vi "Send Initialize DLS Laser.vi"(4 "Fault?":bool, 5 "DLS Status LEDs Refnum":refnum<vi>, 6 "DLS Laser ID (A,B,C or D)":enum16{"A", "B", "C", "D"}(ring), 7 "Priority":T1=enum."Normal" caption="Message Priority (Normal)", 8 "error in (no error)":errorcluster, 9 "DLS Range Refnum":refnum<vi>, 10 "DLS COM Port":refnum<visa-resource-name>, 11 "Message Enqueuer in":refnum<class "Message Enqueuer.lvclass">) -> (0 "error out":errorcluster, 3 "Message Enqueuer out":refnum<class "Message Enqueuer.lvclass">)   [LabVIEW 2018, in "FLS Laser Actor.lvlib" / "Initialize FLS Laser Msg.lvclass"]
doc: "Sends the <b>DLS Laser Actor.lvlib:Initialize DLS Laser Msg.lvclass</b> message.\n\nThis message will call <b>Initialize DLS Laser.vi</b> on the <b>DLS Laser Actor.lvlib:DLS Laser Actor.lvclass</b> actor.\n\n<b>Initialize DLS Laser.vi Description</b>"
uses:
  Initialize FLS Laser Msg.lvclass
  <vilib>/ActorFramework/Message Enqueuer/Message Enqueuer.lvclass
  <vilib>/ActorFramework/Message Enqueuer/Message Priority.ctl
  C:/Program Files (x86)/National Instruments/LabVIEW 2018/vi.lib/ActorFramework/Message/Message.lvclass
  Initialize FLS Laser Msg.lvclass/Initialize FLS Laser Msg.ctl
  <vilib>/ActorFramework/Message Enqueuer/Message Enqueuer.lvclass/Message Enqueuer.ctl
  <vilib>/ActorFramework/Message Priority Queue/Priority Enqueue.vi
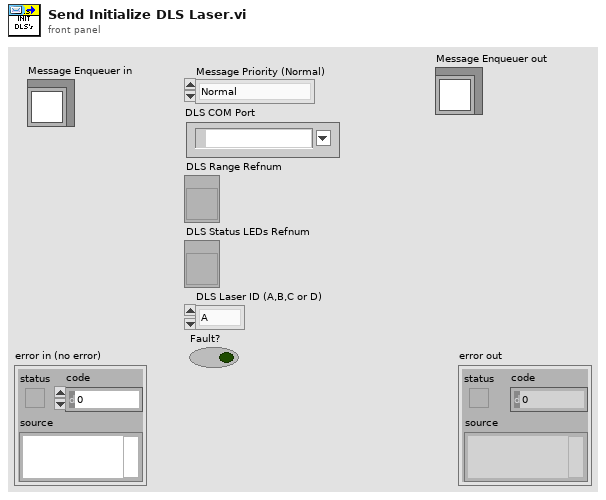
[diagram p1: front panel]
types:
  T1 = typedef "Actor Framework.lvlib/Message Enqueuer.lvclass/Message Priority.ctl" = enum16{"Low", "Normal", "High"}
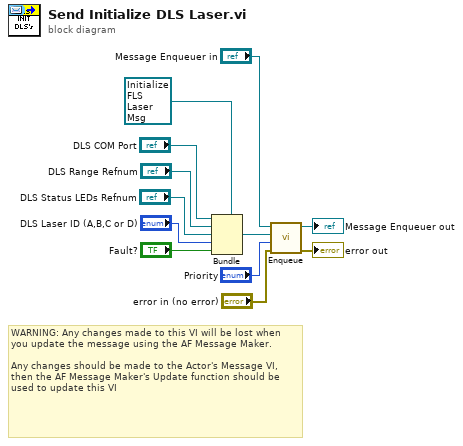
[diagram p0: block diagram]
diagram:
  # "WARNING: Any changes made to this VI will be lost when you update the message using the AF Message Maker.\n\nAny changes should be made to the Actor's Message VI, then the AF Message Maker's Update function should be used to update this VI"
  n1 = Bundle(cluster=refnum<class "Initialize FLS Laser Msg.lvclass"> refnum ("DLS Laser Actor.lvlib:Initialize DLS Laser Msg.lvclass"), "DLS COM Port", "DLS Range Refnum", "DLS Status LEDs Refnum", "DLS Laser ID (A,B,C or D)", "Fault?") -> (w8:refnum<class "Initialize FLS Laser Msg.lvclass">)
  n2 = call <vilib>:"Enqueue.vi"("error in (no error)"="error in (no error)", "Message Priority (Normal)"="Priority", "Message"=w8, "Message Enqueuer in"="Message Enqueuer in") -> ("error out"=→"error out":errorcluster, "Message Enqueuer out"=→"Message Enqueuer out":refnum<class "Message Enqueuer.lvclass">)  [unwired: 6 in]
